vi "GetId.vi"(8 "error in (no error)":errorcluster, 11 "LinkingHeadingId in":refnum<class "LinkingHeadingId.lvclass">) -> (0 "error out":errorcluster, 2 "Id":string, 3 "LinkingHeadingId out":refnum<class "LinkingHeadingId.lvclass">)   [LabVIEW 2021, in "LvMarkdown.lvlib" / "LinkingHeadingId.lvclass"]
uses:
  LinkingHeadingId.lvclass
  LinkingHeadingId.lvclass/LinkingHeadingId.ctl
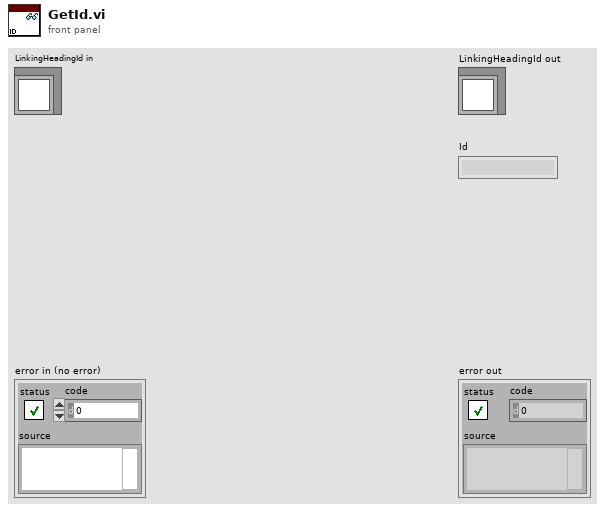
[diagram p1: front panel]
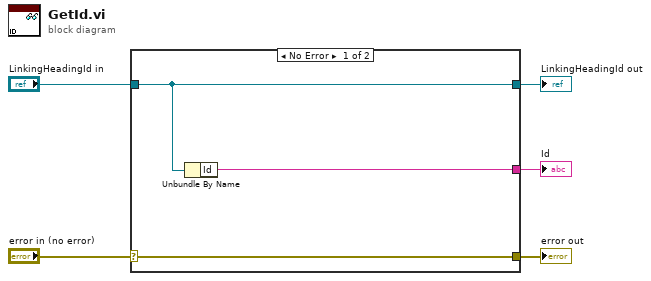
[diagram p0: block diagram]
diagram:
  n1 = case shown="No Error" "error in (no error)" {
    selector: "error in (no error)" -> [w8 w9]
    tunnel: [w8 w9] -> w4
    tunnel: [w7 w10] -> w2
    tunnel: "LinkingHeadingId in" -> [w7 w10]
    tunnel: [w6 _] -> w1
    frame No Error {
      n2 = Unbundle By Name(w7) -> ("Id"=w6:string)
    }
    frame Error {
    }
  }
  "error out" <- w4
  "LinkingHeadingId out" <- w2
  "Id" <- w1
